vi "Flush.vi"(6 "returnNodes":bool, 8 "error in (no error)":errorcluster, 11 "MultiTree in":refnum<class "MultiTree.lvclass">) -> (0 "error out":errorcluster, 2 "Nodes":refnum<data-value>[](array[refnum]), 3 "MultiTree out":refnum<class "MultiTree.lvclass">)   [LabVIEW 2014, in "MultiTree.lvlib" / "MultiTree.lvclass"]
uses:
  <userlib>/AdvancedDataStructures/ClassBased/MultiTree/MultiTree.lvclass
  <userlib>/AdvancedDataStructures/ClassBased/LLNode/LLNode.lvclass
  <userlib>/AdvancedDataStructures/ClassBased/MultiTree/MultiTree.lvclass/MultiTree.ctl
  <userlib>/AdvancedDataStructures/ClassBased/MultiTree/SearchMethod.ctl
  <userlib>/AdvancedDataStructures/ClassBased/MultiTreeNode/MultiTreeNode.lvclass/MultiTreeNode.ctl
  <userlib>/AdvancedDataStructures/ClassBased/MultiTreeNode/MultiTreeNode.lvclass
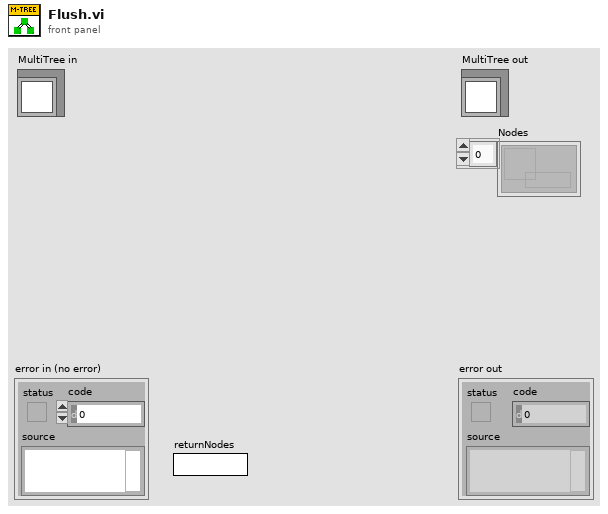
[diagram p1: front panel]
types:
  T1 = typedef "MultiTree.lvlib/MultiTree.lvclass/SearchMethod.ctl" = enum16{"Breadth (First)", "Depth (First)", "Best First", "Breadth (Exhaustive)", "Depth (Exhaustive)"}
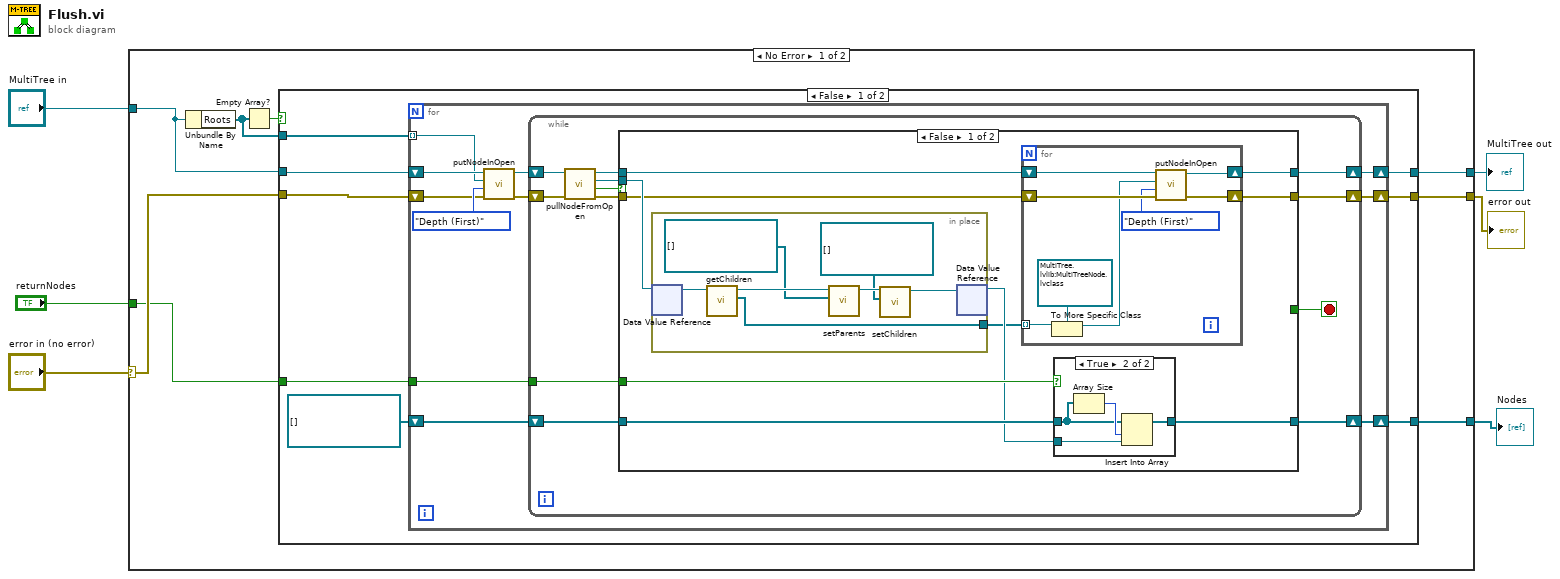
[diagram p0: block diagram]
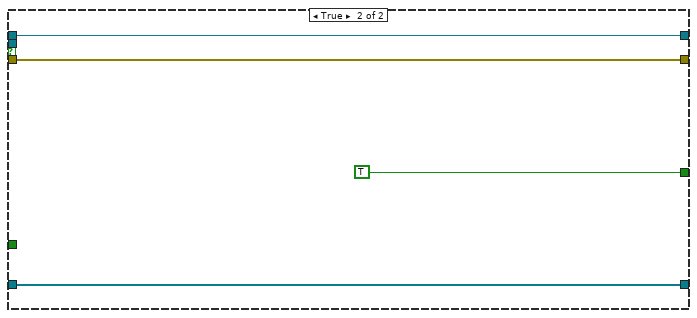
[diagram p3: hidden frame]
diagram:
  n1 = case shown="No Error" "error in (no error)" {
    selector: "error in (no error)" -> [w11 w82]
    tunnel: "MultiTree in" -> [w12 w83]
    tunnel: "returnNodes" -> [w10 _]
    tunnel: [w9 w83] -> w3
    tunnel: [w8 w82] -> w2
    tunnel: [w7 _] -> w1
    frame No Error {
      n2 = Unbundle By Name(w12) -> ("Roots"=w13:refnum<data-value>[])
      n3 = Empty Array?(array=w13) -> (empty?=w14:bool)
      n4 = case shown="False" w14 {
        tunnel: w12 -> [w22 w81]
        tunnel: w13 -> [w21 _]
        tunnel: w11 -> [w20 w80]
        tunnel: w10 -> [w18 _]
        tunnel: [w17 _] -> w7
        tunnel: [w16 w81] -> w9
        tunnel: [w15 w80] -> w8
        frame False {
          n5 = for {
            tunnel: w21 -> [w32] mode=indexing
            tunnel: w18 -> [w26]
            shift-right: [w24] -> w16
            shift-left: w22 -> [w33]
            shift-right: [w23] -> w15
            shift-left: w20 -> [w30]
            shift-right: [w25] -> w17
            shift-left: refnum<data-value>[] [] -> [w27]
            n6 = call <userlib>:"putNodeInOpen.vi"("error in (no error)"=w30, "SearchMethod"=SearchMethod."Depth (First)", "MultiTreeNode"=w32, "MultiTree in"=w33) -> ("error out"=w28:errorcluster, "MultiTree out"=w29:refnum<class "MultiTree.lvclass">)  [unwired: 6 in]
            n7 = while {
              shift-right: [w41] -> w24
              shift-left: w29 -> [w45]
              shift-right: [w39] -> w23
              shift-left: w28 -> [w44]
              shift-right: [w36] -> w25
              shift-left: w27 -> [w37]
              tunnel: w26 -> [w34]
              stop <- w35 stop-if-true
              n8 = call <userlib>:"pullNodeFromOpen.vi"("error in (no error)"=w44, "MultiTree in"=w45) -> ("error out"=w40:errorcluster, "empty"=w43:bool, "RemovedNode"=w38:refnum<data-value>, "MultiTree out"=w42:refnum<class "MultiTree.lvclass">)  [unwired: 6 in]
              n9 = case shown="False" w43 {
                tunnel: w42 -> [w49 w79]
                tunnel: [w47 w79] -> w41
                tunnel: w40 -> [w48 w78]
                tunnel: [w46 w78] -> w39
                tunnel: w38 -> [w55 _]
                tunnel: w37 -> [w53 w77]
                tunnel: [w52 w77] -> w36
                tunnel: [_ TRUE] -> w35
                tunnel: w34 -> [w54 _]
                frame False {
                  n10 = in-place {
                    in-place-border: [w70] -> w50
                    n11 = in-place-dvr #1(w55) -> (w75:refnum<class "MultiTreeNode.lvclass">)  [unwired: 1 out]
                    n12 = call <userlib>:"getChildren.vi"("MultiTreeNode in"=w75) -> ("Children"=w70:refnum<data-value>[], "MultiTreeNode out"=w74:refnum<class "MultiTreeNode.lvclass">)  [unwired: 8 in, 1 out]
                    n13 = call <userlib>:"setParents.vi"("Parents"=refnum<data-value>[] [], "MultiTreeNode in"=w74) -> ("MultiTreeNode out"=w73:refnum<class "MultiTreeNode.lvclass">)  [unwired: 8 in, 1 out]
                    n14 = call <userlib>:"setChildren.vi"("Children"=refnum<data-value>[] [], "MultiTreeNode in"=w73) -> ("MultiTreeNode out"=w71:refnum<class "MultiTreeNode.lvclass">)  [unwired: 8 in, 1 out]
                    n15 = in-place-dvr #1(w71) -> (w51:refnum<data-value>)  [unwired: 1 out]
                  }
                  n16 = for {
                    tunnel: w50 -> [w63] mode=indexing
                    shift-right: [w60] -> w47
                    shift-left: w49 -> [w61]
                    shift-right: [w58] -> w46
                    shift-left: w48 -> [w59]
                    n17 = To More Specific Class(target class=refnum<data-value> refnum ("RemovedNode"), reference=w63) -> (specific class reference=w57:refnum<data-value>)  [unwired: 1 in, 1 out]
                    n18 = call <userlib>:"putNodeInOpen.vi"("error in (no error)"=w59, "SearchMethod"=SearchMethod."Depth (First)", "MultiTreeNode"=w57, "MultiTree in"=w61) -> ("error out"=w58:errorcluster, "MultiTree out"=w60:refnum<class "MultiTree.lvclass">)  [unwired: 6 in]
                  }
                  n19 = case shown="True" w54 {
                    tunnel: w53 -> [w64 w66]
                    tunnel: [w64 w68] -> w52
                    tunnel: w51 -> [_ w65]
                    frame False {
                    }
                    frame True {
                      n20 = Array Size(array=w66) -> (size(s)=w67:i32)
                      n21 = Insert Into Array(array=w66, index=w67, new element=w65) -> (w68:refnum<data-value>[])
                    }
                  }
                }
                frame True {
                }
              }
            }
          }
        }
        frame True {
        }
      }
    }
    frame Error {
    }
  }
  "error out" <- w2
  "MultiTree out" <- w3
  "Nodes" <- w1
